vi "UpdateMode.vi"(8 "error in (no error)":errorcluster, 11 "Instrument in":refnum<class "Instrument.lvclass">) -> (0 "error out":errorcluster, 3 "Instrument out":refnum<class "Instrument.lvclass">)   [LabVIEW 2018, in "Instrument.lvclass"]
uses:
  Instrument.lvclass
  Instrument.lvclass/Instrument.ctl
  Device/Optics/Optics.lvclass/Optics.ctl
  Device/Optics/Opt_Selector/Opt_Selector.lvclass
  C:/Users/devstaff/sparc4/s4gui/Versao ZeroMQ REQ-REP/SPARC4_GUI -v1.0.0 - 20250122_ICS-JSON/Device/Optics/Optics.lvclass
  Device/Optics/Opt_Continuous/Opt_Continuous.lvclass
  StateMachine/State Machine.lvclass
  Device/Optics/Optics.lvclass
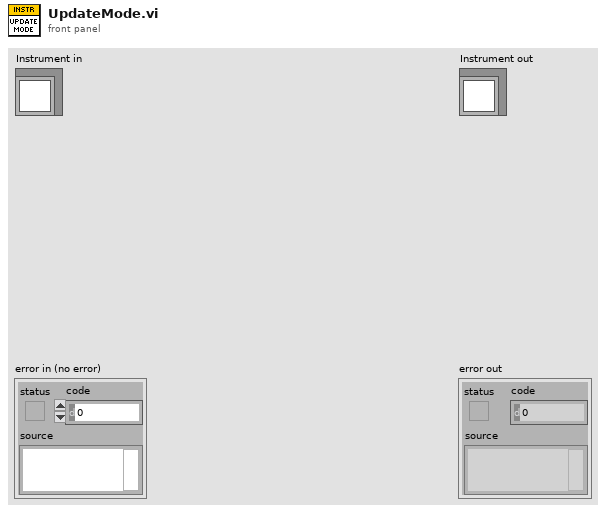
[diagram p1: front panel]
types:
  T1 = cluster{"Photometric":dbl, " Polarimetry":dbl, "Polarimetry \nEfficiency":dbl, "Instrumental polarization":dbl}
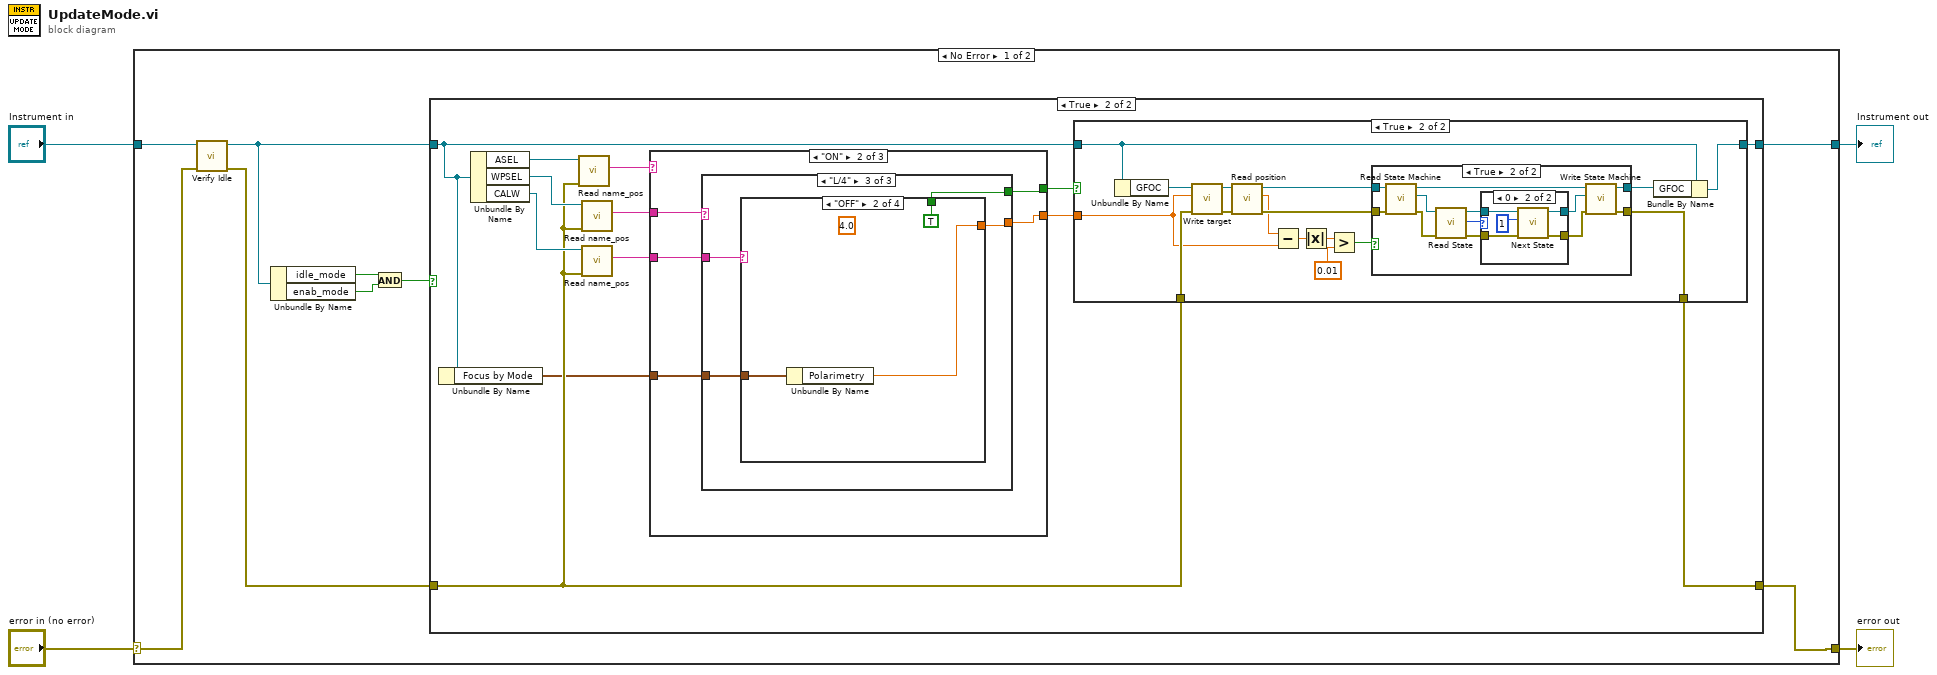
[diagram p0: block diagram]
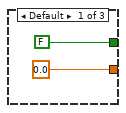
[diagram p6: hidden frame]
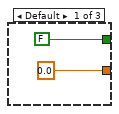
[diagram p7: hidden frame]
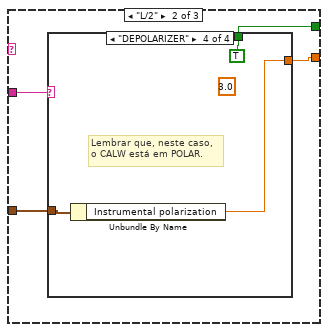
[diagram p8: hidden frame]
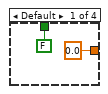
[diagram p9: hidden frame]
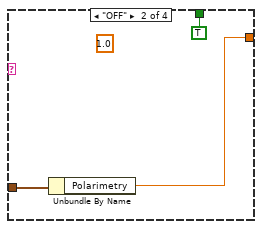
[diagram p10: hidden frame]
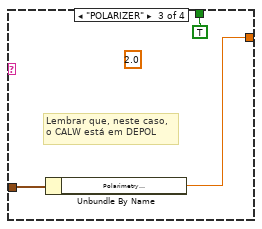
[diagram p11: hidden frame]
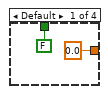
[diagram p12: hidden frame]
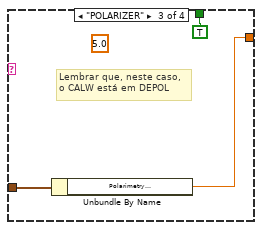
[diagram p13: hidden frame]
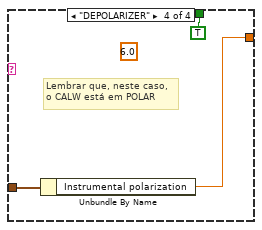
[diagram p14: hidden frame]
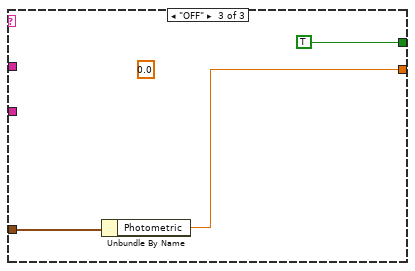
[diagram p15: hidden frame]
diagram:
  n1 = case shown="No Error" "error in (no error)" {
    selector: "error in (no error)" -> [w12 w111]
    tunnel: [w8 w111] -> w3
    tunnel: [w10 w110] -> w1
    tunnel: "Instrument in" -> [w13 w110]
    frame No Error {
      n2 = call-dynamic "Verify Idle.vi"("error in (no error)"=w12, "Instrument in"=w13) -> ("error out"=w9:errorcluster, "Instrument out"=w11:refnum<class "Instrument.lvclass">)  [unwired: 8 in]
      n3 = Unbundle By Name(w11) -> ("idle_mode"=w6:bool, "enab_mode"=w5:bool)
      n4 = And(x=w6, y=w5) -> (x .and. y?=w7:bool)
      n5 = case shown="True" w7 {
        tunnel: w11 -> [w15 w17]
        tunnel: [w15 w22] -> w10
        tunnel: w9 -> [w14 w21]
        tunnel: [w14 w20] -> w8
        frame False {
        }
        frame True {
          n6 = Unbundle By Name(w17) -> ("Focus by Mode"=w16:T1)
          n7 = Unbundle By Name(w17) -> ("ASEL"=w28:refnum<class "Opt_Selector.lvclass">, "WPSEL"=w27:refnum<class "Opt_Selector.lvclass">, "CALW"=w26:refnum<class "Opt_Selector.lvclass">)
          n8 = call "Read name_pos.vi"("error in (no error)"=w21, "Optics in"=w28) -> ("name_pos"=w25:string)  [unwired: 7 in, 2 out]
          n9 = call "Read name_pos.vi"("error in (no error)"=w21, "Optics in"=w27) -> ("name_pos"=w24:string)  [unwired: 7 in, 2 out]
          n10 = call "Read name_pos.vi"("error in (no error)"=w21, "Optics in"=w26) -> ("name_pos"=w23:string)  [unwired: 7 in, 2 out]
          n11 = case shown="\"ON\"" w25 {
            tunnel: w24 -> [_ w74 _]
            tunnel: w23 -> [_ w71 _]
            tunnel: [0.0 w72 w107] -> w18
            tunnel: [FALSE w73 TRUE] -> w19
            tunnel: w16 -> [_ w70 w108]
            frame Default {
            }
            frame "ON" {
              n12 = case shown="\"L/4\"" w74 {
                tunnel: [FALSE w79 w94] -> w73
                tunnel: [0.0 w78 w93] -> w72
                tunnel: w71 -> [_ w80 w95]
                tunnel: w70 -> [_ w77 w92]
                frame Default {
                }
                frame "L/2" {
                  n13 = case shown="\"DEPOLARIZER\"" w80 {
                    tunnel: [FALSE TRUE TRUE TRUE] -> w79
                    tunnel: [0.0 w83 w86 w89] -> w78
                    tunnel: w77 -> [_ w84 w87 w90]
                    frame Default {
                    }
                    frame "OFF" {
                      (unwired) 1.0
                      n14 = Unbundle By Name(w84) -> ("Polarimetry"=w83:dbl)
                    }
                    frame "POLARIZER" {
                      (unwired) 2.0
                      # "Lembrar que, neste caso,\no CALW está em DEPOL"
                      n15 = Unbundle By Name(w87) -> ("Polarimetry \nEfficiency"=w86:dbl)
                    }
                    frame "DEPOLARIZER" {
                      (unwired) 3.0
                      # "Lembrar que, neste caso,\no CALW está em POLAR."
                      n16 = Unbundle By Name(w90) -> ("Instrumental polarization"=w89:dbl)
                    }
                  }
                }
                frame "L/4" {
                  n17 = case shown="\"OFF\"" w95 {
                    tunnel: [FALSE TRUE TRUE TRUE] -> w94
                    tunnel: [0.0 w98 w101 w104] -> w93
                    tunnel: w92 -> [_ w99 w102 w105]
                    frame Default {
                    }
                    frame "OFF" {
                      (unwired) 4.0
                      n18 = Unbundle By Name(w99) -> ("Polarimetry"=w98:dbl)
                    }
                    frame "POLARIZER" {
                      (unwired) 5.0
                      # "Lembrar que, neste caso,\no CALW está em DEPOL"
                      n19 = Unbundle By Name(w102) -> ("Polarimetry \nEfficiency"=w101:dbl)
                    }
                    frame "DEPOLARIZER" {
                      (unwired) 6.0
                      # "Lembrar que, neste caso,\no CALW está em POLAR"
                      n20 = Unbundle By Name(w105) -> ("Instrumental polarization"=w104:dbl)
                    }
                  }
                }
              }
            }
            frame "OFF" {
              (unwired) 0.0
              n21 = Unbundle By Name(w108) -> ("Photometric"=w107:dbl)
            }
          }
          n22 = case shown="True" w19 {
            tunnel: w17 -> [w30 w46]
            tunnel: [w30 w45] -> w22
            tunnel: w21 -> [w29 w43]
            tunnel: [w29 w42] -> w20
            tunnel: w18 -> [_ w35]
            frame False {
            }
            frame True {
              n23 = Unbundle By Name(w46) -> ("GFOC"=w44:refnum<class "Opt_Continuous.lvclass">)
              n24 = call "Write target.vi"("error in (no error)"=w43, "target"=w35, "Optics in"=w44) -> ("error out"=w39:errorcluster, "Optics out"=w40:refnum<class "Opt_Continuous.lvclass">)  [unwired: 7 in]
              n25 = call "Read position.vi"("error in (no error)"=w39, "Optics in"=w40) -> ("error out"=w37:errorcluster, "position"=w36:dbl, "Optics out"=w38:refnum<class "Opt_Continuous.lvclass">)  [unwired: 7 in]
              n26 = Subtract(x=w36, y=w35) -> (x-y=w33:dbl)
              n27 = Absolute Value(x=w33) -> (abs(x)=w31:dbl)
              n28 = Greater?(x=w31, y=0.01) -> (0:w34:bool)
              n29 = case shown="True" w34 {
                tunnel: [w47 w57] -> w42
                tunnel: [w48 w56] -> w41
                tunnel: w38 -> [w48 w55]
                tunnel: w37 -> [w47 w54]
                frame False {
                }
                frame True {
                  n30 = call-dynamic "Read State Machine.vi"("error in (no error)"=w54, "Device in"=w55) -> ("error out"=w49:errorcluster, "State Machine.lvclass"=w50:refnum<class "State Machine.lvclass">, "Device out"=w58:refnum<class "Opt_Continuous.lvclass">)  [unwired: 7 in]
                  n31 = call-dynamic "Read State.vi"("error in (no error)"=w49, "State Machine in"=w50) -> ("error out"=w51:errorcluster, "State"=w53:i32, "State Machine out"=w52:refnum<class "State Machine.lvclass">)  [unwired: 7 in]
                  n32 = case shown="0" w53 {
                    tunnel: [w61 w67] -> w60
                    tunnel: [w62 w66] -> w59
                    tunnel: w52 -> [w62 w64]
                    tunnel: w51 -> [w61 w63]
                    frame Default {
                    }
                    frame 0 {
                      n33 = call "Next State.vi"("error in (no error)"=w63, "New_State"=1, "State Machine in"=w64) -> ("error out"=w67:errorcluster, "State Machine out"=w66:refnum<class "State Machine.lvclass">)  [unwired: 7 in]
                    }
                  }
                  n34 = call-dynamic "Write State Machine.vi"("error in (no error)"=w60, "State Machine.lvclass"=w59, "Device in"=w58) -> ("error out"=w57:errorcluster, "Device out"=w56:refnum<class "Opt_Continuous.lvclass">)  [unwired: 7 in]
                }
              }
              n35 = Bundle By Name(cluster=w46, "GFOC"=w41) -> (w45:refnum<class "Instrument.lvclass">)
            }
          }
        }
      }
    }
    frame Error {
    }
  }
  "error out" <- w3
  "Instrument out" <- w1
